vi "GettingStartedWithLabView.vi"() -> ()   [LabVIEW 2019]
panel:
  in  "stop":bool
  out "Waveform Graph":dynamicdata(graph)
  in  "Amplitude":dbl(knob) scale=0.0..10.0
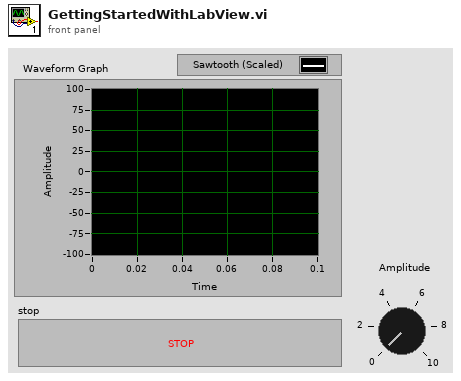
[diagram p1: front panel]
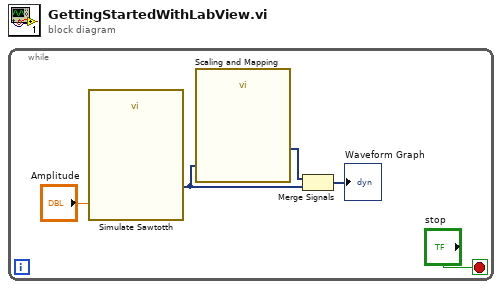
[diagram p0: block diagram]
diagram:
  n1 = while {
    stop <- "stop" stop-if-true
    n2 = call "Simulate Sawtotth"("Amplitude"="Amplitude") -> ("Sawtooth"=w4:dynamicdata)  [unwired: 13 in, 1 out]
    n3 = call "Scaling and Mapping"("Signals"=w4) -> ("Scaled Signals"=w5:dynamicdata)  [unwired: 9 in, 1 out]
    n4 = Merge Signals(w5, w4) -> (→"Waveform Graph":dynamicdata)
  }
